vi "Location Possible.vi"(8 "error in (no error)":errorcluster, 9 "Target":refnum<vi>, 10 "Desired Location":dbl[](array[numeric]), 11 "Data In":T1={"link 1 angle"=0.0, "link 2 angle"=0.0, "link 1 length"=0.0, "link 2 length"=0.0, "Current arm location"=[{"X"=0.0, "Y"=0.0}, {"X"=-37.249783598972314, "Y"=33.353464914904016}, {"X"=-74.49956719794463, "Y"=66.70692982980803}], "Link Picture"=bytes[1162], "Desired Location"={"Desired X"=0.0, "Desired Y"=0.0}, "Next Location"={"Next X"=0.0, "Next Y"=0.0}, "Error"={"Joint1 error"=0.0, "Joint2 error"=0.0}, "tdms data"=refnum, "de/dt"={"joint1 de/dt"=0.0, "joint2 de/dt"=0.0}, "Voltages"={"Joint1 voltage"=0.0, "Joint2 voltage"=0.0}, "Time"=0.0, "dt"=0.0, "counts/rev"=0.0, "kp"=0.0, "kd"=0.0, "ki"=0.0, "Int(error)"={"joint1 int(e)"=0.0, "joint2 int(e)"=0.0}, "Desired angles"={"theta 1"=0.0, "theta 2"=0.0}, "Current counts"={"theta 1"=0.0, "theta 2"=0.0}, "Desired Counts"={"theta 1"=0.0, "theta 2"=0.0}, "Preivous Error"={"Joint1 Previous error"=0.0, "Joint2 Previous error"=0.0}, "Counts/s"=0.0, "Correct counter"=0}) -> (0 "error out":errorcluster, 3 "Data Out":T1={"link 1 angle"=0.0, "link 2 angle"=0.0, "link 1 length"=0.0, "link 2 length"=0.0, "Current arm location"=[{"X"=0.0, "Y"=0.0}, {"X"=-37.249783598972314, "Y"=33.353464914904016}, {"X"=-74.49956719794463, "Y"=66.70692982980803}], "Link Picture"=bytes[1162], "Desired Location"={"Desired X"=0.0, "Desired Y"=0.0}, "Next Location"={"Next X"=0.0, "Next Y"=0.0}, "Error"={"Joint1 error"=0.0, "Joint2 error"=0.0}, "tdms data"=refnum, "de/dt"={"joint1 de/dt"=0.0, "joint2 de/dt"=0.0}, "Voltages"={"Joint1 voltage"=0.0, "Joint2 voltage"=0.0}, "Time"=0.0, "dt"=0.0, "counts/rev"=0.0, "kp"=0.0, "kd"=0.0, "ki"=0.0, "Int(error)"={"joint1 int(e)"=0.0, "joint2 int(e)"=0.0}, "Desired angles"={"theta 1"=0.0, "theta 2"=0.0}, "Current counts"={"theta 1"=0.0, "theta 2"=0.0}, "Desired Counts"={"theta 1"=0.0, "theta 2"=0.0}, "Preivous Error"={"Joint1 Previous error"=0.0, "Joint2 Previous error"=0.0}, "Counts/s"=0.0, "Correct counter"=0})   [LabVIEW 2017]
doc: "This VI whether the desired location is physically possible by comparing the maximum extended length of the arm with the desired distance from the origin.\n\nIf the desired location is possible then the desired location will be updated. If the desired location is impossible then it will not be updated."
uses:
  Type Defs/Host Data.ctl
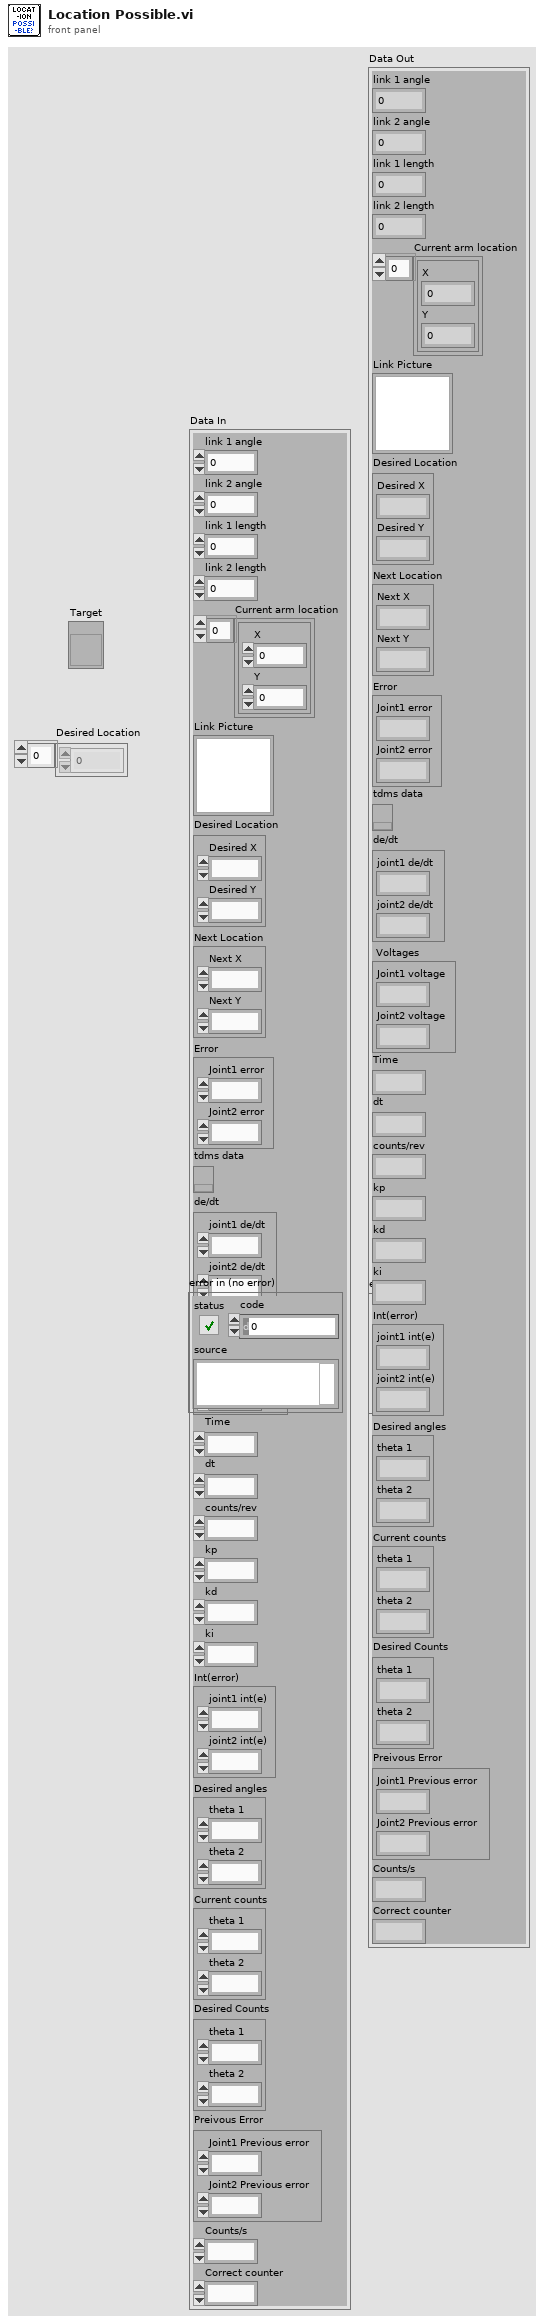
[diagram p1: front panel]
types:
  T1 = typedef "Host Data.ctl" = cluster{"link 1 angle":dbl, "link 2 angle":dbl, "link 1 length":dbl, "link 2 length":dbl, "Current arm location":cluster{"X":dbl, "Y":dbl}[], "Link Picture":picture, "Desired Location":cluster{"Desired X":dbl, "Desired Y":dbl}, "Next Location":cluster{"Next X":dbl, "Next Y":dbl}, "Error":cluster{"Joint1 error":dbl, "Joint2 error":dbl}, "tdms data":refnum<k34>, "de/dt":cluster{"joint1 de/dt":dbl, "joint2 de/dt":dbl}, "Voltages":cluster{"Joint1 voltage":dbl, "Joint2 voltage":dbl}, "Time":dbl, "dt":dbl, "counts/rev":dbl, "kp":dbl, "kd":dbl, "ki":dbl, "Int(error)":cluster{"joint1 int(e)":dbl, "joint2 int(e)":dbl}, "Desired angles":cluster{"theta 1":dbl, "theta 2":dbl}, "Current counts":cluster{"theta 1":dbl, "theta 2":dbl}, "Desired Counts":cluster{"theta 1":dbl, "theta 2":dbl}, "Preivous Error":cluster{"Joint1 Previous error":dbl, "Joint2 Previous error":dbl}, "Counts/s":dbl, "Correct counter":i32}
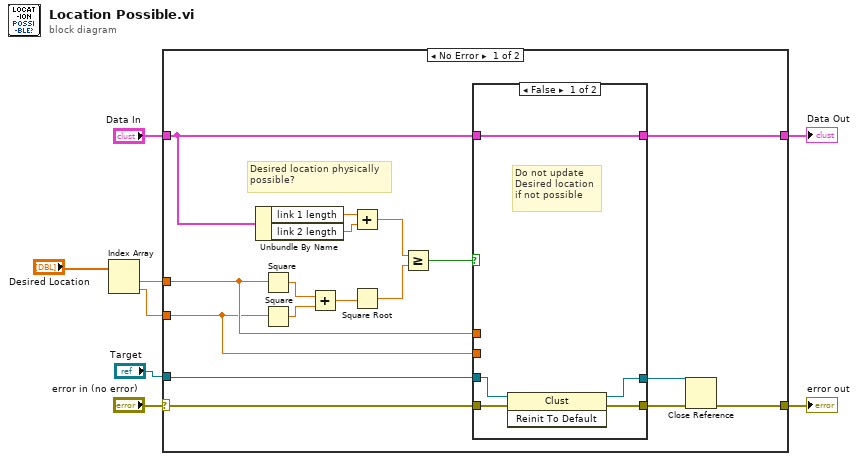
[diagram p0: block diagram]
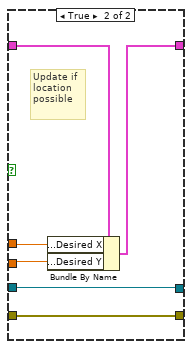
[diagram p2: hidden frame]
diagram:
  n1 = Index Array(array="Desired Location") -> (element #1=w3:dbl, element #2=w1:dbl)  [unwired: 2 in]
  n2 = case shown="No Error" "error in (no error)" {
    selector: "error in (no error)" -> [w12 w38]
    tunnel: [w10 w38] -> w7
    tunnel: "Data In" -> [w15 w37]
    tunnel: w3 -> [w17 _]
    tunnel: w1 -> [w16 _]
    tunnel: [w14 w37] -> w5
    tunnel: "Target" -> [w13 _]
    frame No Error {
      # "Desired location physically\npossible?"
      n3 = Unbundle By Name(w15) -> ("link 1 length"=w24:dbl, "link 2 length"=w25:dbl)
      n4 = Square(x=w17) -> (x^2=w23:dbl)
      n5 = Square(x=w16) -> (x^2=w22:dbl)
      n6 = Add(x=w23, y=w22) -> (x+y=w21:dbl)
      n7 = Add(x=w24, y=w25) -> (x+y=w20:dbl)
      n8 = Square Root(x=w21) -> (sqrt(x)=w19:dbl)
      n9 = Greater Or Equal?(x=w20, y=w19) -> (x >= y?=w18:bool)
      n10 = case shown="False" w18 {
        tunnel: w17 -> [_ w35]
        tunnel: w16 -> [_ w34]
        tunnel: w15 -> [w30 w36]
        tunnel: [w30 w33] -> w14
        tunnel: w13 -> [w29 w31]
        tunnel: w12 -> [w27 w32]
        tunnel: [w28 w32] -> w11
        tunnel: [w26 w31] -> w9
        frame False {
          # "Do not update\nDesired location\nif not possible"
          n11 = invoke class="Clust" method="Reinit To Default"(reference=w29, error in=w27) -> (reference out=w26:refnum<vi>, error out=w28:errorcluster)  [unwired: 1 in, 1 out]
        }
        frame True {
          # "Update if location possible"
          n12 = Bundle By Name(cluster=w36, "Desired Location.Desired X"=w35, "Desired Location.Desired Y"=w34) -> (w33:T1)
        }
      }
      n13 = Close Reference(reference=w9, error in (no error)=w11) -> (error out=w10:errorcluster)
    }
    frame Error {
    }
  }
  "error out" <- w7
  "Data Out" <- w5
